vi "Teleop.vi"(10 "Match Info":T1={"Autonomous Elapsed Seconds"=0.0, "TeleOp Elapsed Seconds"=0.0, "Disabled Elapsed Seconds"=0.0, "Visited Autonomous"=FALSE, "Visited TeleOp"=FALSE, "Visited Disabled"=FALSE, "Autonomous Settings"={"Autonomous Style"=enum."Independent", "VI Refnum"=refnum}}, 11 "Call Context":T2) -> ()   [LabVIEW 2016]
doc: "This VI is called for each enabled TeleOp packet received from the DS. It is typically used to read from joysticks and other inputs and update I/O or setpoints for timed control loops. It should complete and return within 20 milliseconds or risk missing DS packets."
uses:
  <vilib>/Rock Robotics/WPI/DriverStation/WPI_DriverStationDerivedRobotMode.ctl
  <vilib>/Rock Robotics/WPI/DriverStation/WPI_DriverStationMatch Info.ctl
  <vilib>/Rock Robotics/WPI/Utilities/WPI_GetSetVariantRefNum.vi
  <vilib>/Rock Robotics/Network Tables/NT Write Boolean Array.vi
  <vilib>/Rock Robotics/Network Tables/NT Write Numeric Array.vi
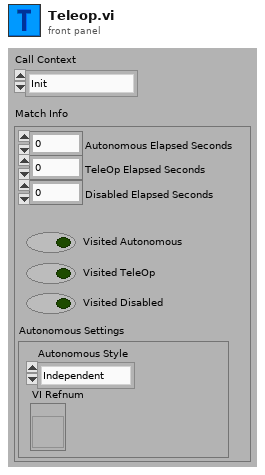
[diagram p1: front panel]
types:
  T1 = typedef "WPI_DriverStationMatch Info.ctl" = cluster{"Autonomous Elapsed Seconds":dbl, "TeleOp Elapsed Seconds":dbl, "Disabled Elapsed Seconds":dbl, "Visited Autonomous":bool, "Visited TeleOp":bool, "Visited Disabled":bool, "Autonomous Settings":cluster{"Autonomous Style":enum16{"Iterative", "Independent"}, "VI Refnum":refnum<vi>}}
  T2 = typedef "WPI_DriverStationDerivedRobotMode.ctl" = enum16{"Init", "Execute", "Stop"}
  T3 = typedef "WPI_JoystickDevRef.ctl" = cluster{"Device":T4}
  T4 = typedef "WPI_JoystickDeviceEnum.ctl" = enum16{"USB 0", "USB 1", "USB 2", "USB 3", "USB 4", "USB 5"}
  T5 = typedef "Command Status Info.ctl" = cluster{"Name":string, "Status":T6, "notifier out":T7}
  T6 = typedef "Completion Status.ctl" = enum16{"Successful", "Aborted", "Incomplete"}
  T7 = typedef "Completion Notifier.ctl" = refnum<notifier>
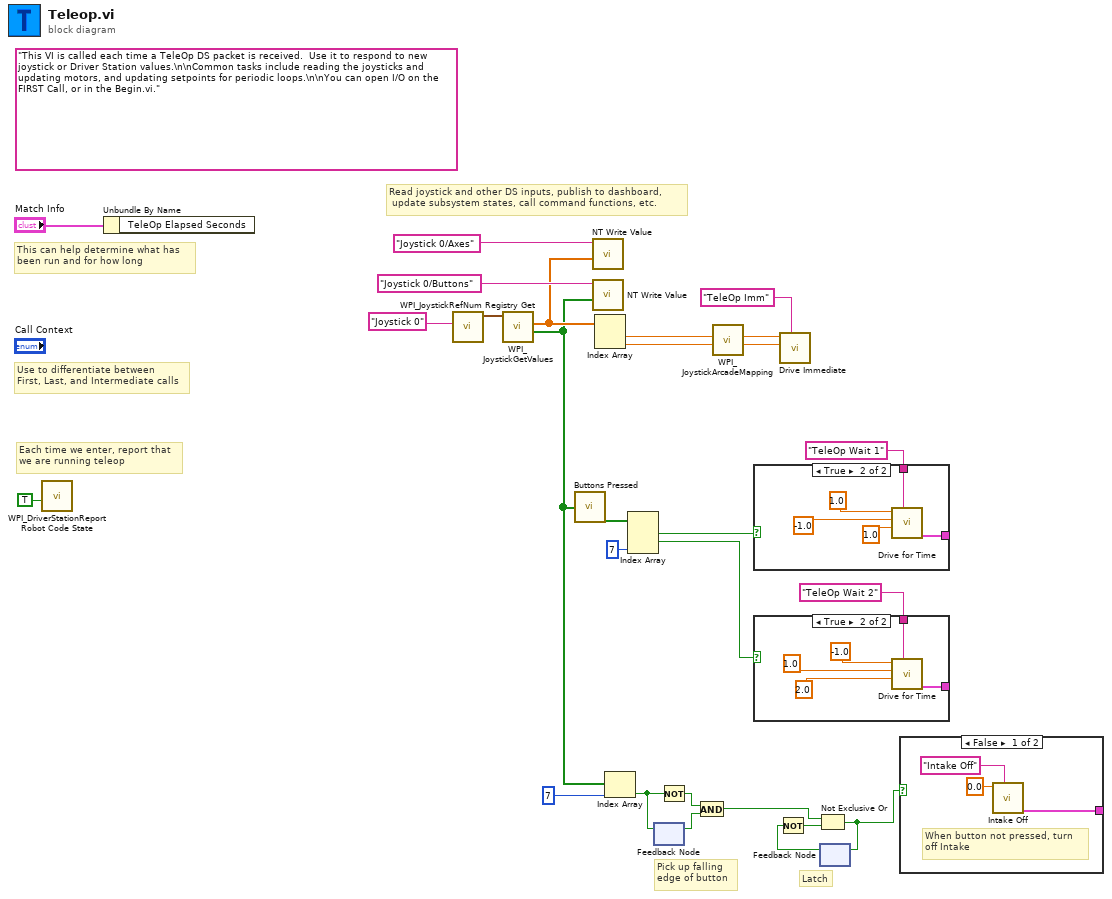
[diagram p0: block diagram]
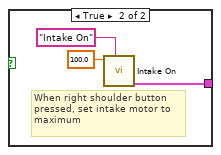
[diagram p2: hidden frame]
diagram:
  (unwired) "This VI is called each time a TeleOp DS packet is received.  Use it to respond to new joystick or Driver Station values.\n\nCommon tasks include reading the joysticks and updating motors, and updating setpoints for periodic loops.\n\nYou can open I/O on the FIRST Call, or in the Begin.vi."
  # "Latch"
  # "Pick up falling\nedge of button"
  # "Read joystick and other DS inputs, publish to dashboard,\n update subsystem states, call command functions, etc."
  # "Each time we enter, report that\nwe are running teleop"
  # "Use to differentiate between\nFirst, Last, and Intermediate calls"
  # "This can help determine what has\nbeen run and for how long"
  n1 = call <vilib>:"WPI_DriverStationReport Robot Code State.vi"("TeleOp"=TRUE ("Autonomous")) -> ()  [unwired: 10 in, 1 out]
  n2 = Unbundle By Name("Match Info") -> ()  [unwired: 1 out]
  n3 = call <vilib>:"WPI_JoystickRefNum Registry Get.vi"("refnum name"="Joystick 0") -> ("JoystickDevRef"=w24:T3)  [unwired: 1 in, 9 out]
  n4 = call <vilib>:"WPI_JoystickGetValues.vi"("JoystickDevRef"=w24) -> ("Buttons"=w9:bool[], "Axes"=w12:dbl[])  [unwired: 6 in, 3 out]
  n5 = call "Buttons Pressed.vi"("Button Values"=w9) -> ("Button Presses"=w20:bool[])
  n6 = call-poly <vilib>:"NT Write Value.vi"("Numeric Array"=w12, "Name"="Joystick 0/Axes") -> ()  [unwired: 9 in, 1 out]
  n7 = call-poly <vilib>:"NT Write Value.vi"("Boolean Array"=w9, "Name"="Joystick 0/Buttons") -> ()  [unwired: 9 in, 1 out]
  n8 = Index Array(array=w12) -> (element #1=w15:dbl, element #2=w14:dbl)  [unwired: 2 in]
  n9 = Index Array(array=w9, index=7) -> (element=w7:bool)
  n10 = Index Array(array=w20, index #3=7 ("index")) -> (element #1=w19:bool, element #2=w18:bool)  [unwired: 2 in, 1 out]
  n11 = feedback-in #1(w7) -> ()
  n12 = feedback #1() -> (w5:bool)  [unwired: 1 in]
  n13 = Not(x=w7) -> (.not. x?=w6:bool)
  n14 = And(x=w6, y=w5) -> (x .and. y?=w3:bool)
  n15 = call <vilib>:"WPI_JoystickArcadeMapping.vi"("Y axis value"=w14, "X axis value"=w15) -> ("Right Motor Value"=w16:dbl, "Left Motor Value"=w17:dbl)  [unwired: 8 in]
  n16 = case shown="True" w19 {
    tunnel: [_ w31] -> _
    tunnel: "TeleOp Wait 1" ("Description") -> [_ w30]
    frame False {
    }
    frame True {
      n17 = call "Drive for Time.vi"("Description"=w30, "Seconds"=1.0, "Right Speed"=-1.0, "Left Speed"=1.0) -> ("Command Info Out"=w31:T5)  [unwired: 6 in, 1 out]
    }
  }
  n18 = case shown="True" w18 {
    tunnel: [_ w35] -> _
    tunnel: "TeleOp Wait 2" ("Description") -> [_ w34]
    frame False {
    }
    frame True {
      n19 = call "Drive for Time.vi"("Description"=w34, "Seconds"=2.0, "Right Speed"=1.0, "Left Speed"=-1.0) -> ("Command Info Out"=w35:T5)  [unwired: 6 in, 1 out]
    }
  }
  n20 = call "Drive Immediate.vi"("Description"="TeleOp Imm", "Right Setpoint"=w16, "Left Setpoint"=w17) -> ()  [unwired: 8 in, 1 out]
  n21 = feedback #2() -> (w2:bool)  [unwired: 1 in]
  n22 = Not(x=w2) -> (.not. x?=w4:bool)
  n23 = Not Exclusive Or(1:w4, 2:w3) -> (0:w1:bool)
  n24 = feedback-in #2(w1) -> ()
  n25 = case shown="False" w1 {
    tunnel: [w39 w42] -> _
    frame False {
      # "When button not pressed, turn\noff Intake"
      n26 = call "Intake Off.vi"("Description"="Intake Off", "Setpoint"=0.0) -> ("Command Info Out"=w39:T5)  [unwired: 9 in]
    }
    frame True {
      # "When right shoulder button \npressed, set intake motor to \nmaximum"
      n27 = call "Intake On.vi"("Description"="Intake On", "Setpoint"=100.0) -> ("Command Info Out"=w42:T5)  [unwired: 9 in]
    }
  }
